vi "QuerySystemHW.vi"(8 "error in (no error)":errorcluster) -> (0 "error out":errorcluster)   [LabVIEW 2017, in "SystemInfoProcess.lvlib"]
doc: "Checks the status of system hardware."
uses:
  <vilib>/addons/SystemInfoProcess/SystemInfoProcess.lvlib
  <vilib>/addons/PointValueMap/subVIs/Point_Write_variant.vi
  <vilib>/addons/cRIODetectHW/cRIODetectHW.lvlib
  <vilib>/addons/PointValueMap/PointValueMap.lvlib
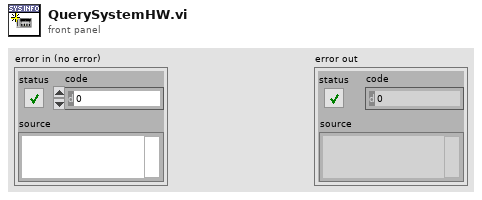
[diagram p1: front panel]
types:
  T1 = typedef "PointValueMap.lvlib/PointMap.ctl" = refnum<data-value>
  T2 = typedef "cRIODetectHW.lvlib/SystemHW.ctl" = cluster{"controller":T3, "chassis":T3, "modules":T3[]}
  T3 = typedef "cRIODetectHW.lvlib/cRIO Product Info.ctl" = cluster{"vendorName":string, "productName":string, "serialNumber":string}
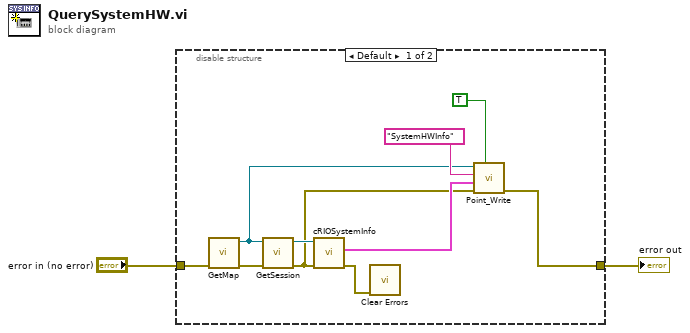
[diagram p0: block diagram]
diagram:
  n1 = disable-structure shown="Default" {
    disable-tunnel: "error in (no error)" -> [w7 w13]
    disable-tunnel: [w12 w13] -> w1
    frame condition #0 (active) {
      n2 = call <vilib>:"GetMap.vi"("error in (no error)"=w7) -> ("error out"=w8:errorcluster, "SystemInfoMap"=w5:T1)  [unwired: 9 in]
      n3 = call <vilib>:"GetSession.vi"("error in (no error)"=w8, "map"=w5) -> ("error out"=w4:errorcluster, "session"=w6:refnum<k21>)  [unwired: 8 in]
      n4 = call <vilib>:"cRIOSystemInfo.vi"("error in (no error)"=w4, "session in"=w6) -> ("error out"=w3:errorcluster, "system info"=w10:T2)  [unwired: 8 in]
      n5 = call <vilib>:"Clear Errors.vi"("error in (no error)"=w3) -> ()  [unwired: 5 in, 2 out]
      n6 = call-poly <vilib>:"Point_Write.vi"("Auto Create?"=TRUE, "Error In"=w4, "Value"=w10, "Tag"="SystemHWInfo", "Map"=w5) -> ("Error Out"=w12:errorcluster)  [unwired: 5 in, 1 out]
    }
    frame condition #1 {
    }
  }
  "error out" <- w1
